vi "FTS Get Acquisition Option Auto Gain.vi"(8 "error in (no error)":errorcluster, 11 "specIndex":u16) -> (0 "error out":errorcluster, 3 "function return":bool)   [LabVIEW 2010, in "FTSLib.lvlib"]
doc: "bool __cdecl FTS_GetAcquisitionOption_AutoGain(unsigned short specIndex);"
uses:
  FTSLib.lvlib
  FTSLib.dll
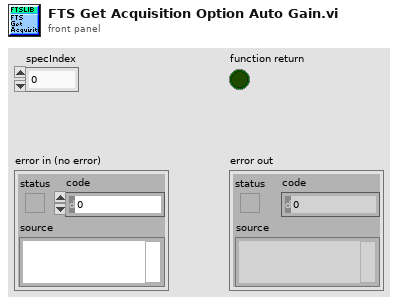
[diagram p1: front panel]
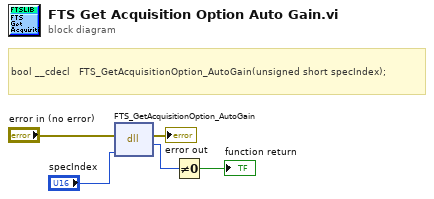
[diagram p0: block diagram]
diagram:
  # "bool __cdecl   FTS_GetAcquisitionOption_AutoGain(unsigned short specIndex);"
  n1 = dll-call lib="FTSLib.*" fn="FTS_GetAcquisitionOption_AutoGain"(error in="error in (no error)", "specIndex"="specIndex") -> (error out=→"error out":errorcluster, w4:u8)  [unwired: 3 in, 1 out]
  n2 = Not Equal To 0?(x=w4) -> (x != 0?=→"function return":bool)
